vi "List of error rings.vi"   [LabVIEW 2016]
uses:
  <vilib>/Utility/error.llb/Error Cluster From Error Code.vi
  <vilib>/ErrorRing/Error Ring.xnode
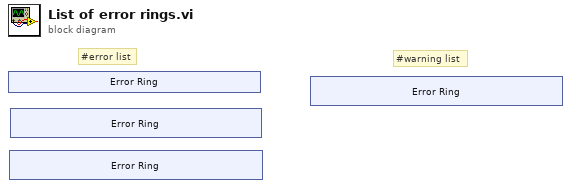
[diagram p0: block diagram]
diagram:
  # "#warning list"
  # "#error list"
  n1 = xnode "Error Ring"() -> ()  [unwired: 1 out]
  n2 = xnode "Error Ring"() -> ()  [unwired: 1 in, 1 out]
  n3 = xnode "Error Ring"() -> ()  [unwired: 1 in, 1 out]
  n4 = xnode "Error Ring"() -> ()  [unwired: 1 in, 1 out]
